vi "datatrimmer.vi"(8 "max x":dbl=1.0, 9 "min x":dbl=1.0, 10 "y":dbl[](array[numeric]), 11 "x":dbl[](array[numeric])) -> (2 "trimmed y":dbl[](array[numeric]), 3 "trimmed x":dbl[](array[numeric]))   [LabVIEW 2020]
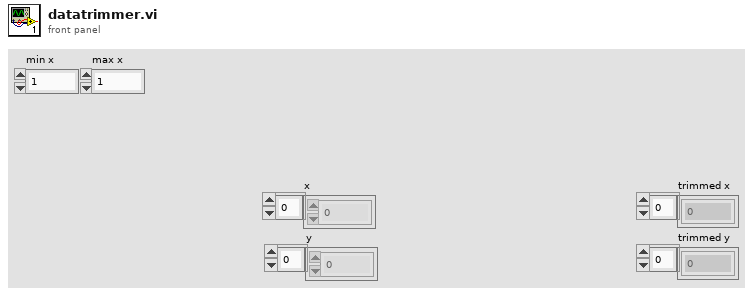
[diagram p1: front panel]
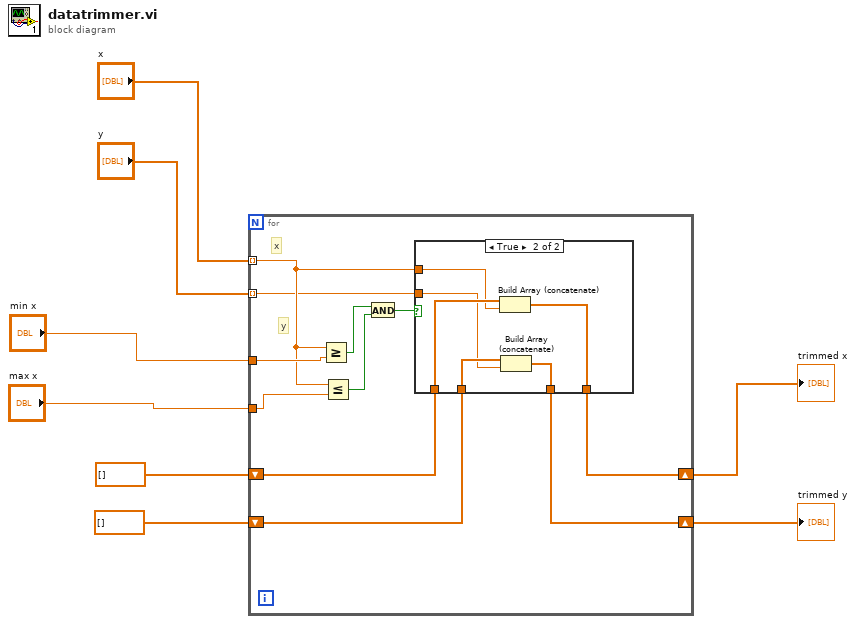
[diagram p0: block diagram]
diagram:
  n1 = for {
    tunnel: "x" -> [w14] mode=indexing
    tunnel: "y" -> [w13] mode=indexing
    tunnel: "min x" -> [w18]
    tunnel: "max x" -> [w17]
    shift-right: [w10] -> w2
    shift-left: dbl[] [] -> [w12]
    shift-right: [w9] -> w1
    shift-left: dbl[] [] -> [w11]
    # "y"
    # "x"
    n2 = Greater Or Equal?(x=w14, y=w18) -> (x >= y?=w16:bool)
    n3 = Less Or Equal?(x=w14, y=w17) -> (x <= y?=w15:bool)
    n4 = And(x=w16, y=w15) -> (x .and. y?=w19:bool)
    n5 = case shown="True" w19 {
      tunnel: w14 -> [_ w25]
      tunnel: w13 -> [_ w24]
      tunnel: w12 -> [w21 w27]
      tunnel: w11 -> [w20 w26]
      tunnel: [w21 w23] -> w10
      tunnel: [w20 w22] -> w9
      frame False {
      }
      frame True {
        n6 = Build Array (concatenate)(w27, w25) -> (w23:dbl[])
        n7 = Build Array (concatenate)(w26, w24) -> (w22:dbl[])
      }
    }
  }
  "trimmed x" <- w2
  "trimmed y" <- w1
